vi "sub_vi_calibration.vi"(8 "error in (no error)":errorcluster, 10 "Gain":u16, 11 "VISA resource name":refnum<visa-resource-name>) -> (0 "error out":errorcluster, 1 "Weights":dbl[](array[numeric]), 2 "Measures":dbl[](array[numeric]), 3 "VISA resource name out":refnum<visa-resource-name>, 4 "Relative errors array":dbl[](array[numeric]), 5 "Calibration - read data":dbl[][](array[numeric]), 6 "Absolute errors array":dbl[](array[numeric]), 7 "Noise":dbl)   [LabVIEW 2019]
uses:
  <vilib>/Analysis/baseanly.llb/Mean (DBL).vi
  <vilib>/Analysis/NI_AALBase.lvlib
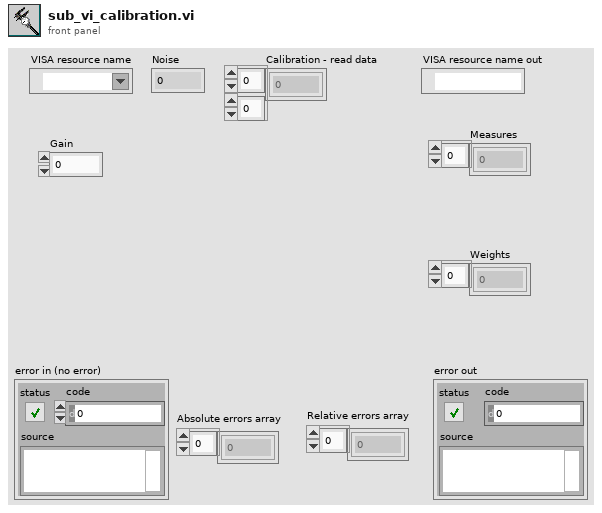
[diagram p1: front panel]
types:
  T1 = cluster{"[0]":dbl, "[1]":dbl, "[2]":dbl, "[3]":dbl, "[4]":dbl, "[5]":dbl, "[6]":dbl, "[7]":dbl, "[8]":dbl}
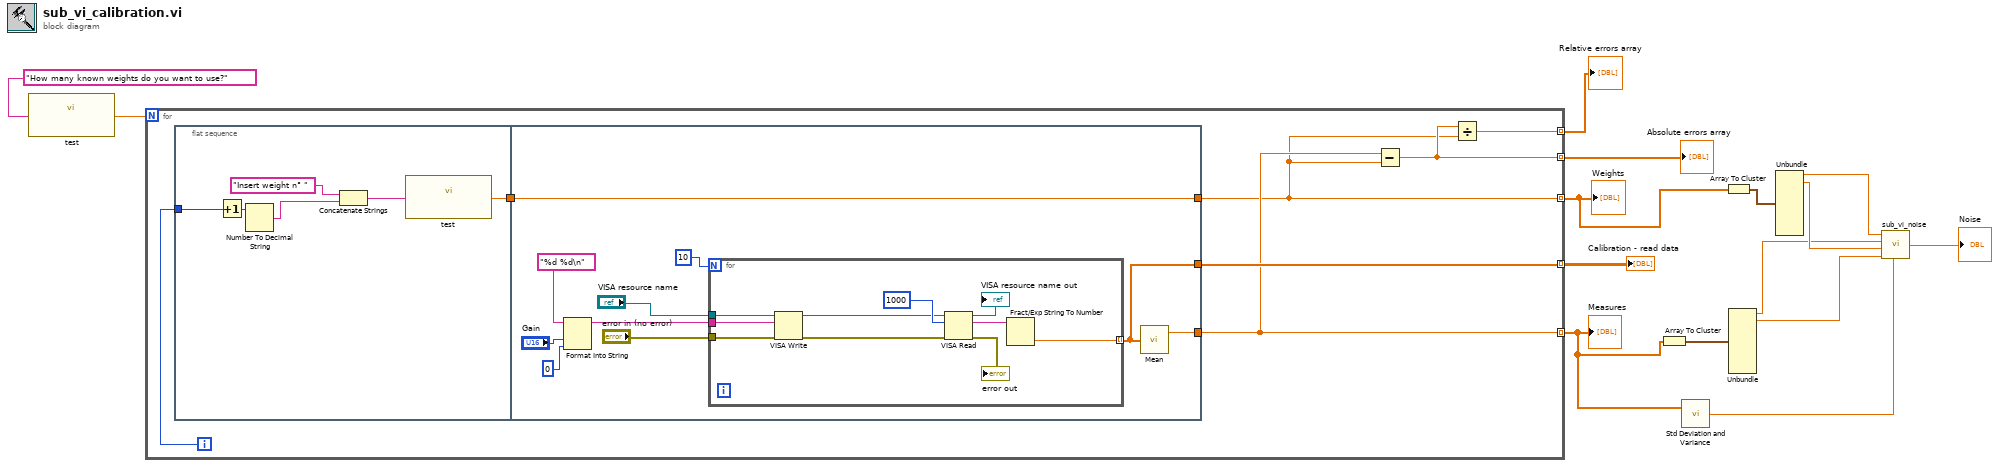
[diagram p0: block diagram]
diagram:
  n1 = call "test.vi"("Title"="How many known weights do you want to use?") -> ("Weights number 2"=w14:dbl)  [unwired: 18 in]
  n2 = for {
    N: w14 -> [_]
    tunnel: [w17] -> w10 mode=indexing
    tunnel: [w19] -> w3 mode=indexing
    tunnel: [w20] -> w13 mode=indexing
    tunnel: [w18] -> w12 mode=indexing
    tunnel: [w16] -> w11 mode=indexing
    i -> [w22]
    n3 = flat-sequence {
      tunnel: w22 -> [w25]
      tunnel: [w23] -> w21
      tunnel: [w38] -> w17
      tunnel: w21 -> [w38]
      tunnel: [w33] -> w19
      tunnel: [w29] -> w20
      frame #0 {
        n4 = Increment(x=w25) -> (x+1=w28:i32)
        n5 = Number To Decimal String(number=w28) -> (decimal integer string=w27:string)  [unwired: 1 in]
        n6 = Concatenate Strings("Insert weight n° ", w27) -> (w26:string)
        n7 = call "test.vi"("Title"=w26) -> ("Weights number 2"=w23:dbl)  [unwired: 18 in]
      }
      frame #1 {
        n8 = Format Into String(format string="%d %d\n", "Gain", u16 0 ("input 2")) -> (resulting string=w31:string)  [unwired: 2 in, 1 out]
        n9 = for {
          N: 10 -> [_]
          tunnel: [w44] -> w29 mode=indexing
          tunnel: "error in (no error)" -> [w43]
          tunnel: w31 -> [w42]
          tunnel: "VISA resource name" -> [w41]
          n10 = VISA Write(VISA resource name=w41, write buffer=w42, error in (no error)=w43) -> (VISA resource name out=w39:refnum<visa-resource-name>, error out=w40:errorcluster)  [unwired: 1 out]
          n11 = VISA Read(VISA resource name=w39, byte count=u32 1000, error in (no error)=w40) -> (VISA resource name out=→"VISA resource name out":refnum<visa-resource-name>, read buffer=w47:string, error out=→"error out":errorcluster)  [unwired: 1 out]
          n12 = Fract/Exp String To Number(string=w47) -> (number=w44:dbl)  [unwired: 3 in, 1 out]
        }
        n13 = call-poly <vilib>:"Mean.vi"("X"=w29) -> ("mean"=w33:dbl)  [unwired: 1 out]
      }
    }
    n14 = Subtract(x=w19, y=w17) -> (x-y=w18:dbl)
    n15 = Divide(x=w18, y=w17) -> (x/y=w16:dbl)
  }
  "Weights" <- w10
  "Measures" <- w3
  "Calibration - read data" <- w13
  "Absolute errors array" <- w12
  "Relative errors array" <- w11
  n16 = Array To Cluster(array=w3) -> (cluster=w6:T1)
  n17 = call <vilib>:"Std Deviation and Variance.vi"("X"=w3) -> ("standard deviation"=w2:dbl)  [unwired: 1 in, 2 out]
  n18 = Array To Cluster(array=w10) -> (cluster=w9:T1)
  n19 = Unbundle(w6) -> ("[0]"=w5:dbl, "[1]"=w4:dbl)  [unwired: 7 out]
  n20 = Unbundle(w9) -> ("[0]"=w8:dbl, "[1]"=w7:dbl)  [unwired: 7 out]
  n21 = call "sub_vi_noise.vi"("x1"=w8, "y1"=w5, "x2"=w7, "sigma"=w2, "y2"=w4) -> ("Noise"=→"Noise":dbl)  [unwired: 3 in]
